vi "Stop Core.vi"(10 "final error code":i32, 11 "Single Assert Display in":refnum<class "Single Assert Display.lvclass">) -> (3 "Single Assert Display out":refnum<class "Single Assert Display.lvclass">)   [LabVIEW 2016, in "Assert API Components.lvlib" / "Assert Display.lvlib" / "Single Assert Display.lvlib" / "Single Assert Display.lvclass"]
doc: "(<B>Filename</B>: Actor Framework.lvlib:Actor.lvclass:Stop Core.vi)\n\nDefines what the actor does before it stops. Use the <B>final error code</B> input to determine whether the actor shut down in response to an error.\n\nBy default, this method does nothing. A descendant class may override it to define behavior, such as shutting down any processes the actor initiated in its override of the Actor Core method."
uses:
  Single Assert Display.lvclass
  Single Assert Display.lvclass/Single Assert Display.ctl
  Base UI Actor/Base UI Actor/Base UI Actor.lvclass
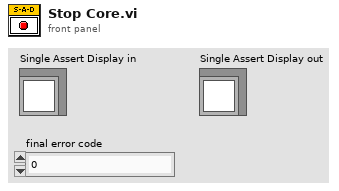
[diagram p1: front panel]
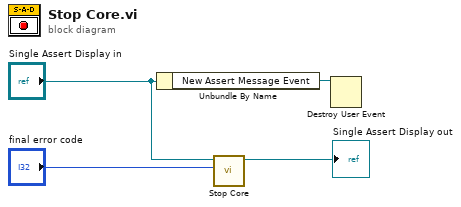
[diagram p0: block diagram]
diagram:
  n1 = Unbundle By Name("Single Assert Display in") -> ("New Assert Message Event"=w1:refnum<user-event>)
  n2 = call-parent "Stop Core.vi"("final error code"="final error code", "Base UI Actor in"="Single Assert Display in") -> ("Base UI Actor out"=→"Single Assert Display out":refnum<class "Single Assert Display.lvclass">)  [unwired: 9 in]
  n3 = Destroy User Event(user event=w1) -> ()  [unwired: 1 in, 1 out]
